vi "Handle Response.vi"(7 "Processing In":refnum<class "Processing.lvclass">, 11 "Authentication Handler in":refnum<class "Authentication Handler.lvclass">) -> (0 "error out":errorcluster, 5 "Processing":refnum<class "Processing.lvclass">)   [LabVIEW 2020, in "HTTP Server.lvlib" / "Authentication Handler.lvclass"]
uses:
  Authentication Handler.lvclass
  Processing/Processing.lvclass/Processing.ctl
  lv-http-util/HTTP Utils/Request/Request.lvclass/Request.ctl
  lv-uri/URI/URI/URI.lvclass/URI.ctl
  lv-uri/URI/URI/Path String.vi
  lv-uri/URI/Build URI String.vi
  lv-uri/URI/Build Query String.vi
  Authentication Handler.lvclass/Authentication Handler.ctl
  Processing/Processing.lvclass
  Authentication Provider/Authentication Provider.lvclass
  Security/Security.lvclass
  lv-http-util/HTTP Utils/Method.ctl
  lv-http-util/HTTP Utils/HTTP Utils.lvlib
  lv-http-util/HTTP Utils/Request/Request.lvclass
  lv-uri/URI/URI/URI.lvclass
  Session/Session.lvclass
  Values/Values.lvclass
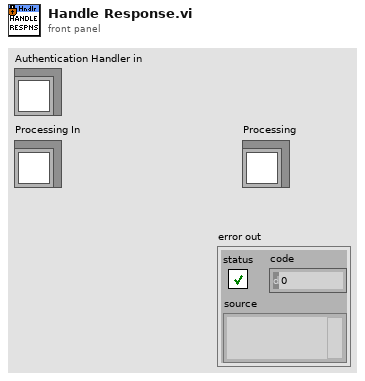
[diagram p1: front panel]
types:
  T1 = typedef "HTTP Utils.lvlib/Method.ctl" = enum16{"GET", "HEAD", "POST", "PUT", "DELETE", "CONNECT", "OPTIONS", "TRACE", "PATCH"}
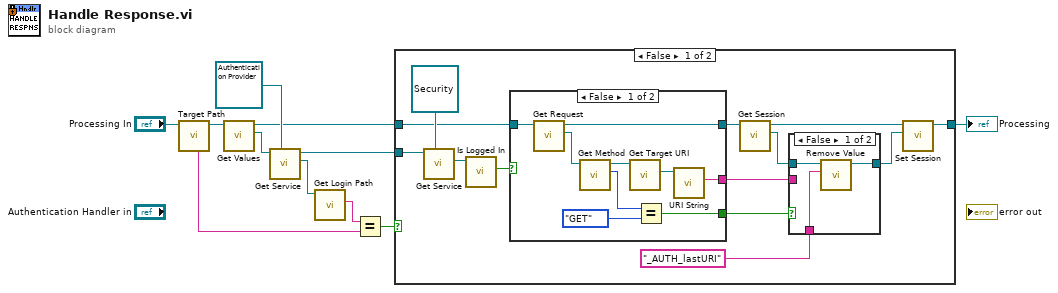
[diagram p0: block diagram]
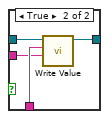
[diagram p2: hidden frame]
diagram:
  n1 = call "Target Path.vi"("Processing in"="Processing In") -> ("Processing out"=w4:refnum<class "Processing.lvclass">, "Target Path"=w2:string)  [unwired: 9 in]
  n2 = call "Get Values.vi"("Processing in"=w4) -> ("Values"=w10:refnum<class "Values.lvclass">, "Processing out"=w7:refnum<class "Processing.lvclass">)  [unwired: 9 in]
  n3 = call "Get Service.vi"("Service Type"=refnum<class "Authentication Provider.lvclass"> refnum ("HTTP Server.lvlib:Authentication Provider.lvclass"), "Values in"=w10) -> ("Service"=w6:refnum<class "Authentication Provider.lvclass">, "Values out"=w8:refnum<class "Values.lvclass">)  [unwired: 7 in, 1 out]
  n4 = call-dynamic "Get Login Path.vi"("Authentication Provider in"=w6) -> ("Login Path"=w3:string)  [unwired: 8 in, 2 out]
  n5 = Equal?(x=w3, y=w2) -> (x = y?=w1:bool)
  n6 = case shown="False" w1 {
    tunnel: [w16 w42] -> w11
    tunnel: w8 -> [w15 _]
    tunnel: w7 -> [w12 w42]
    frame False {
      n7 = call "Get Service.vi"("Service Type"=refnum<class "Security.lvclass"> refnum ("HTTP Server.lvlib:Security.lvclass"), "Values in"=w15) -> ("Service"=w13:refnum<class "Security.lvclass">)  [unwired: 7 in, 2 out]
      n8 = call "Is Logged In.vi"("Security in"=w13) -> ("Logged In"=w24:bool)  [unwired: 8 in, 2 out]
      n9 = case shown="False" w24 {
        tunnel: w12 -> [w40 w41]
        tunnel: [w33 _] -> w22
        tunnel: [w36 _] -> w21
        tunnel: [w32 w41] -> w23
        frame False {
          n10 = call "Get Request.vi"("Processing in"=w40) -> ("Request"=w39:refnum<class "Request.lvclass">, "Processing out"=w32:refnum<class "Processing.lvclass">)  [unwired: 9 in]
          n11 = call "Get Method.vi"("Request in"=w39) -> ("Method"=w35:T1, "Request out"=w38:refnum<class "Request.lvclass">)  [unwired: 8 in, 1 out]
          n12 = call "Get Target URI.vi"("Request in"=w38) -> ("Target URI"=w37:refnum<class "URI.lvclass">)  [unwired: 8 in, 2 out]
          n13 = Equal?(x=w35, y=Method."GET") -> (x = y?=w33:bool)
          n14 = call "URI String.vi"("URI in"=w37) -> ("URI String"=w36:string)  [unwired: 9 in, 1 out]
        }
        frame True {
        }
      }
      n15 = call "Get Session.vi"("Processing in"=w23) -> ("Session"=w20:refnum<class "Session.lvclass">, "Processing out"=w18:refnum<class "Processing.lvclass">)  [unwired: 9 in]
      n16 = case shown="False" w22 {
        tunnel: w21 -> [_ w29]
        tunnel: w20 -> [w27 w31]
        tunnel: "_AUTH_lastURI" -> [w26 w30]
        tunnel: [w25 w28] -> w17
        frame False {
          n17 = call "Remove Value.vi"("Name"=w26, "Session in"=w27) -> ("Session out"=w25:refnum<class "Session.lvclass">)  [unwired: 6 in, 3 out]
        }
        frame True {
          n18 = call "Write Value.vi"("Value"=w29, "Name"=w30, "Session in"=w31) -> ("Session out"=w28:refnum<class "Session.lvclass">)  [unwired: 6 in, 2 out]
        }
      }
      n19 = call "Set Session.vi"("Session"=w17, "Processing in"=w18) -> ("Processing out"=w16:refnum<class "Processing.lvclass">)  [unwired: 9 in]
    }
    frame True {
      # "Don't update path if on the configured login path"
    }
  }
  "Processing" <- w11
